vi "Update UI Status String.vi"(8 "error in (no error)":errorcluster, 10 "Status":string, 11 "Test Application Controller in":refnum<class "Test Application Controller.lvclass">) -> (0 "error out":errorcluster, 3 "Test Application Controller out":refnum<class "Test Application Controller.lvclass">)   [LabVIEW 2017, in "Test Application Controller.lvlib" / "Test Application Controller.lvclass"]
uses:
  Test Application Controller.lvclass
  Test Application Controller.lvclass/Test Application Controller.ctl
  User Interface Messages/Update Status String Msg/Update Status String Msg.lvclass/Update Status String Msg.ctl
  <vilib>/ActorFramework/Message Enqueuer/Message Enqueuer.lvclass/Message Enqueuer.ctl
  <vilib>/ActorFramework/Message Enqueuer/Enqueue.vi
  User Interface Messages/Update Status String Msg/Update Status String Msg.lvclass
  C:/Program Files (x86)/National Instruments/LabVIEW 2017/vi.lib/ActorFramework/Message/Message.lvclass
  <vilib>/ActorFramework/Message Priority Queue/Priority Enqueue.vi
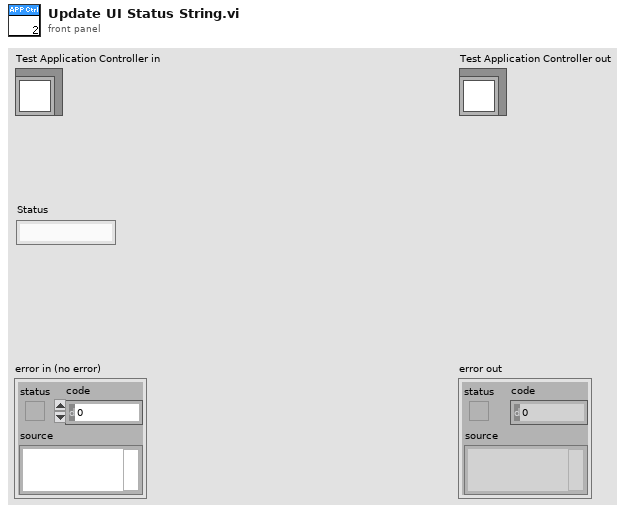
[diagram p1: front panel]
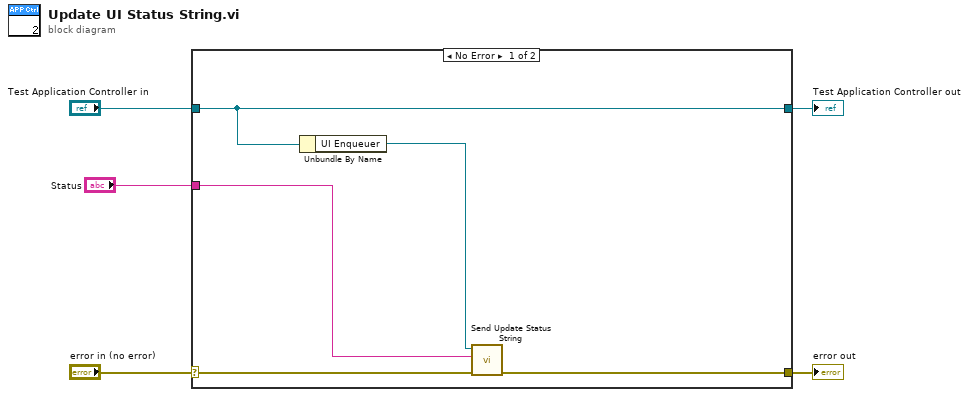
[diagram p0: block diagram]
diagram:
  n1 = case shown="No Error" "error in (no error)" {
    selector: "error in (no error)" -> [w9 w12]
    tunnel: [w6 w12] -> w4
    tunnel: [w10 w11] -> w2
    tunnel: "Test Application Controller in" -> [w10 w11]
    tunnel: "Status" -> [w7 _]
    frame No Error {
      n2 = Unbundle By Name(w10) -> ("UI Enqueuer"=w8:refnum<class "Message Enqueuer.lvclass">)
      n3 = call "Send Update Status String.vi"("error in (no error)"=w9, "Status"=w7, "Message Enqueuer"=w8) -> ("error out"=w6:errorcluster)  [unwired: 7 in, 1 out]
    }
    frame Error {
    }
  }
  "error out" <- w4
  "Test Application Controller out" <- w2
